vi "2283_drive.vi"(0 "Auto-Aim":bool, 1 "Invert":bool, 2 "Gyro Angle":dbl, 3 "Axes[1]":dbl, 4 "Axis[4]":dbl, 5 "Numeric Array":dbl[](array[numeric])) -> (14 "Motor Izquierdo":dbl, 19 "Motor Derecho":dbl)   [LabVIEW 2015]
uses:
  <vilib>/addons/control/pid/pid.llb/PID Lead-Lag (DBL).vi
  <vilib>/addons/control/pid/pid.llb/PID (DBL).vi
  <vilib>/addons/control/pid/NI_PID_pid.lvlib
panel:
  in  "Max Output":dbl=1.0
  in  "tuning parameters giro":T1={"gain"=1.0, "lag time"=0.01, "lead time"=0.0} {"lead time" format="%.3f"; "lag time" format="%.3f"; "gain" format="%.3f"}
  in  "tuning parameters":T1={"gain"=1.0, "lag time"=0.15, "lead time"=0.0} {"lead time" format="%.3f"; "lag time" format="%.3f"; "gain" format="%.3f"}
  in  "output range":cluster{"output high":dbl, "output low":dbl}={"output high"=1.0, "output low"=-1.0} {"output low" format="%.2f"; "output high" format="%.2f"}
  in  "dt (s)":dbl=-1.0 format="%.3f"
  in  "PID gains":T2={"proportional gain (Kc)"=1.0, "integral time (Ti, min)"=0.052, "derivative time (Td, min)"=0.02} {"derivative time (Td, min)" format="%.3f"; "integral time (Ti, min)" format="%.3f"; "proportional gain (Kc)" format="%.3f"}
  out "Waveform Chart":dbl(graph)
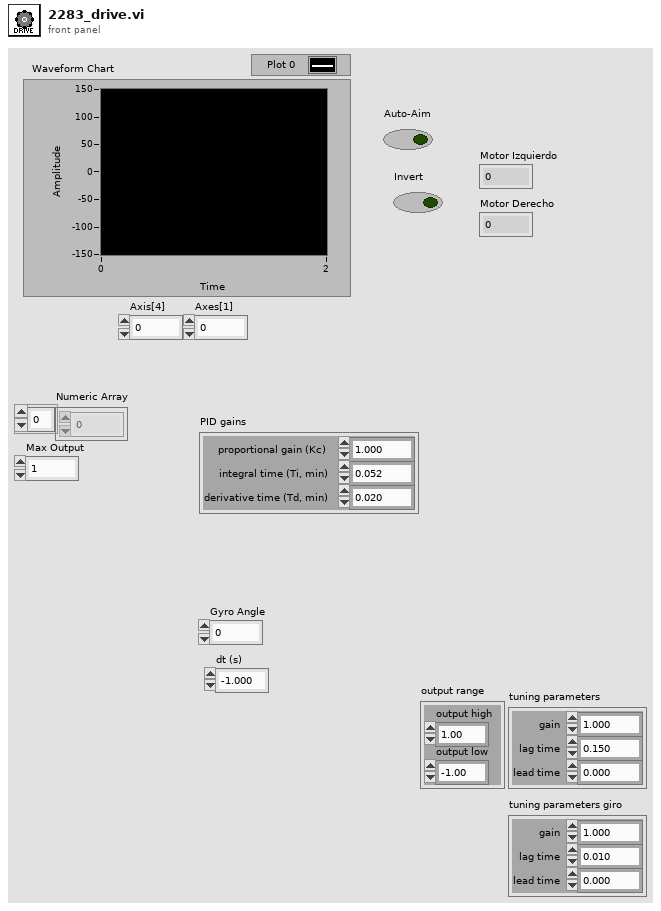
[diagram p1: front panel]
types:
  T1 = cluster{"gain":dbl, "lag time":dbl, "lead time":dbl}
  T2 = cluster{"proportional gain (Kc)":dbl, "integral time (Ti, min)":dbl, "derivative time (Td, min)":dbl}
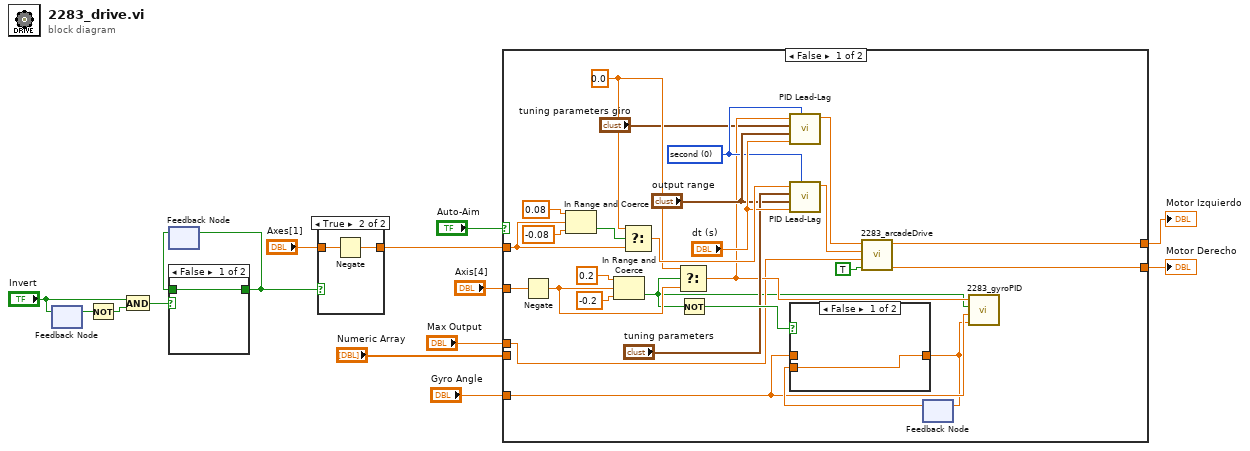
[diagram p0: block diagram]
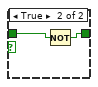
[diagram p2: hidden frame]
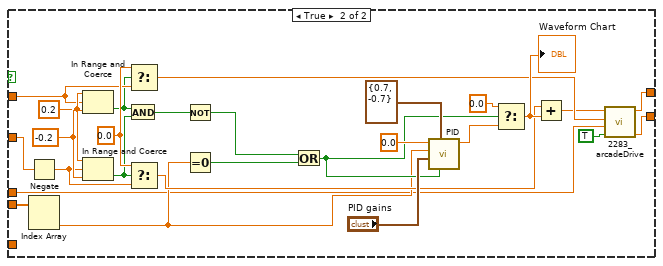
[diagram p5: hidden frame]
diagram:
  n1 = feedback #1() -> (w13:bool)  [unwired: 1 in]
  n2 = feedback-in #1("Invert") -> ()
  n3 = Not(x=w13) -> (.not. x?=w12:bool)
  n4 = And(x="Invert", y=w12) -> (x .and. y?=w8:bool)
  n5 = feedback #2() -> (w7:bool)  [unwired: 1 in]
  n6 = case shown="False" w8 {
    tunnel: [w16 w18] -> w6
    tunnel: w7 -> [w16 w17]
    frame False {
    }
    frame True {
      n7 = Not(x=w17) -> (.not. x?=w18:bool)
    }
  }
  n8 = feedback-in #2(w6) -> ()
  n9 = case shown="True" w6 {
    tunnel: [w19 w20] -> w10
    tunnel: "Axes[1]" -> [w19 w21]
    frame False {
    }
    frame True {
      n10 = Negate(x=w21) -> (-x=w20:dbl)
    }
  }
  n11 = case shown="False" "Auto-Aim" {
    tunnel: w10 -> [w43 w61]
    tunnel: "Axis[4]" -> [w48 w62]
    tunnel: [w29 w58] -> w1
    tunnel: [w28 w57] -> w2
    tunnel: "Gyro Angle" -> [w31 _]
    tunnel: "Numeric Array" -> [_ w59]
    tunnel: "Max Output" -> [w27 w55]
    frame False {
      w37 = u16 0 items=["second", "minute"] ("time unit")
      w44 = 0.0 ("t")
      n12 = Negate(x=w48) -> (-x=w42:dbl)
      n13 = In Range and Coerce(upper limit=0.08, x=w43, lower limit=-0.08) -> (In Range?=w22:bool)  [unwired: 1 out]
      n14 = In Range and Coerce(upper limit=0.2, x=w42, lower limit=-0.2 ("upper limit")) -> (In Range?=w23:bool)  [unwired: 1 out]
      n15 = Select(t=w44, s=w22, f=w43) -> (s? t:f=w45:dbl)
      n16 = Select(t=w44, s=w23, f=w42) -> (s? t:f=w36:dbl)
      n17 = Not(x=w23) -> (.not. x?=w41:bool)
      n18 = call-poly <vilib>:"PID Lead-Lag.vi"("time unit"=w37, "dt (s)"="dt (s)", "output range"="output range", "tuning parameters"="tuning parameters giro", "input"=w36) -> ("output"=w24:dbl)  [unwired: 3 in, 1 out]
      n19 = call-poly <vilib>:"PID Lead-Lag.vi"("time unit"=w37, "dt (s)"="dt (s)", "output range"="output range", "tuning parameters"="tuning parameters", "input"=w45) -> ("output"=w25:dbl)  [unwired: 3 in, 1 out]
      n20 = call "2283_arcadeDrive.vi"("Square Inputs"=TRUE, "Max Output"=w27, "Y axis value"=w25, "X axis value"=w24) -> ("Right Motor Value"=w28:dbl, "Left Motor Value"=w29:dbl)  [unwired: 6 in]
      n21 = feedback #3() -> (w32:dbl)  [unwired: 1 in]
      n22 = case shown="False" w41 {
        tunnel: w31 -> [_ w50]
        tunnel: [w49 w50] -> w30
        tunnel: w32 -> [w49 _]
        frame False {
        }
        frame True {
        }
      }
      n23 = feedback-in #3(w30) -> ()
      n24 = call "2283_gyroPID.vi"("Y Axis Input"=w36, "Y Input?"=w23, "Angulo Actual"=w31, "Angulo Deseado"=w30) -> ()  [unwired: 1 in, 1 out]
    }
    frame True {
      w65 = 0.0 ("t")
      w67 = -0.2 ("lower limit")
      w66 = 0.2 ("upper limit")
      n25 = Negate(x=w62) -> (-x=w64:dbl)
      n26 = Index Array(array=w59) -> (element #2=w60:dbl)  [unwired: 2 in, 1 out]
      n27 = In Range and Coerce(upper limit=w66, x=w61, lower limit=w67) -> (In Range?=w51:bool)  [unwired: 1 out]
      n28 = In Range and Coerce(upper limit=w66, x=w64, lower limit=w67) -> (In Range?=w52:bool)  [unwired: 1 out]
      n29 = And(x=w51, y=w52) -> (x .and. y?=w74:bool)
      n30 = Select(t=w65, s=w51, f=w61) -> (s? t:f=w54:dbl)
      n31 = Select(t=w65, s=w52, f=w64) -> (s? t:f=w63:dbl)
      n32 = Not(x=w74) -> (.not. x?=w72:bool)
      n33 = Equal To 0?(x=w60) -> (x = 0?=w73:bool)
      n34 = Or(x=w72, y=w73) -> (x .or. y?=w69:bool)
      n35 = call-poly <vilib>:"PID.vi"("reinitialize? (F)"=w69, "output range"=cluster{"output high":dbl, "output low":dbl} {"output high"=0.7, "output low"=-0.7}, "PID gains"="PID gains", "process variable"=w60, "setpoint"=0.0) -> ("output"=w71:dbl)  [unwired: 5 in, 1 out]
      n36 = Select(t=0.0, s=w69, f=w71) -> (s? t:f=w68:dbl)
      "Waveform Chart" <- w68
      n37 = Add(x=w63, y=w68) -> (x+y=w53:dbl)
      n38 = call "2283_arcadeDrive.vi"("Square Inputs"=TRUE, "Max Output"=w55, "Y axis value"=w54, "X axis value"=w53) -> ("Right Motor Value"=w57:dbl, "Left Motor Value"=w58:dbl)  [unwired: 6 in]
    }
  }
  "Motor Izquierdo" <- w1
  "Motor Derecho" <- w2
